vi "Test Assert Greater.vi"(8 "error in (no error)":errorcluster) -> (0 "error out":errorcluster)   [LabVIEW 2009]
uses:
  classes/Assert/Assert.lvclass
  classes/Test/Test.lvclass
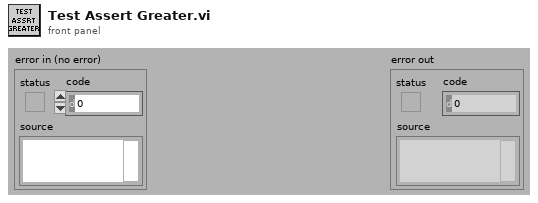
[diagram p1: front panel]
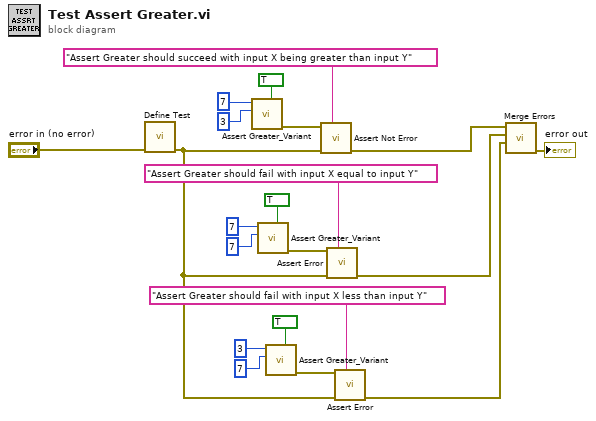
[diagram p0: block diagram]
diagram:
  n1 = call "Define Test.vi"("error in (no error)"="error in (no error)") -> ("error out"=w3:errorcluster)  [unwired: 10 in]
  n2 = call "Assert Greater_Variant.vi"("Assert Only? (F)"=TRUE, "Y"=3, "X"=7) -> ("error out"=w21:errorcluster)  [unwired: 8 in]
  n3 = call "Assert Greater_Variant.vi"("Assert Only? (F)"=TRUE, "Y"=7, "X"=7) -> ("error out"=w19:errorcluster)  [unwired: 8 in]
  n4 = call "Assert Greater_Variant.vi"("Assert Only? (F)"=TRUE, "Y"=7, "X"=3) -> ("error out"=w8:errorcluster)  [unwired: 8 in]
  n5 = call "Assert Not Error.vi"("Label"="Assert Greater should succeed with input X being greater than input Y", "error in (no error)"=w3, "Not Error?"=w21) -> ("error out"=w14:errorcluster)  [unwired: 8 in]
  n6 = call "Assert Error.vi"("Label"="Assert Greater should fail with input X equal to input Y", "error in (no error)"=w3, "Error?"=w19) -> ("error out"=w2:errorcluster)  [unwired: 8 in]
  n7 = call "Assert Error.vi"("Label"="Assert Greater should fail with input X less than input Y", "error in (no error)"=w3, "Error?"=w8) -> ("error out"=w1:errorcluster)  [unwired: 8 in]
  n8 = call <vilib>:"Merge Errors.vi"("error in 3 (no error)"=w1, "error in 2 (no error)"=w2, "error in 1 (no error)"=w14) -> ("error out"=→"error out":errorcluster)  [unwired: 4 in]
